vi "sprawdzanie.vi"(5 "String":string, 6 "String 2":string, 7 "String 6":string, 8 "String 3":string, 9 "String 7":string, 10 "String 4":string, 11 "String 8":string, 12 "String 5":string, 13 "String 9":string) -> (18 "X or O":bool, 19 "String 10":string)   [LabVIEW 2023]
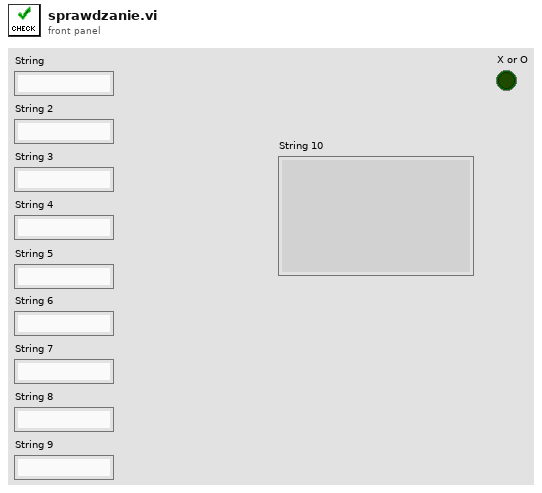
[diagram p1: front panel]
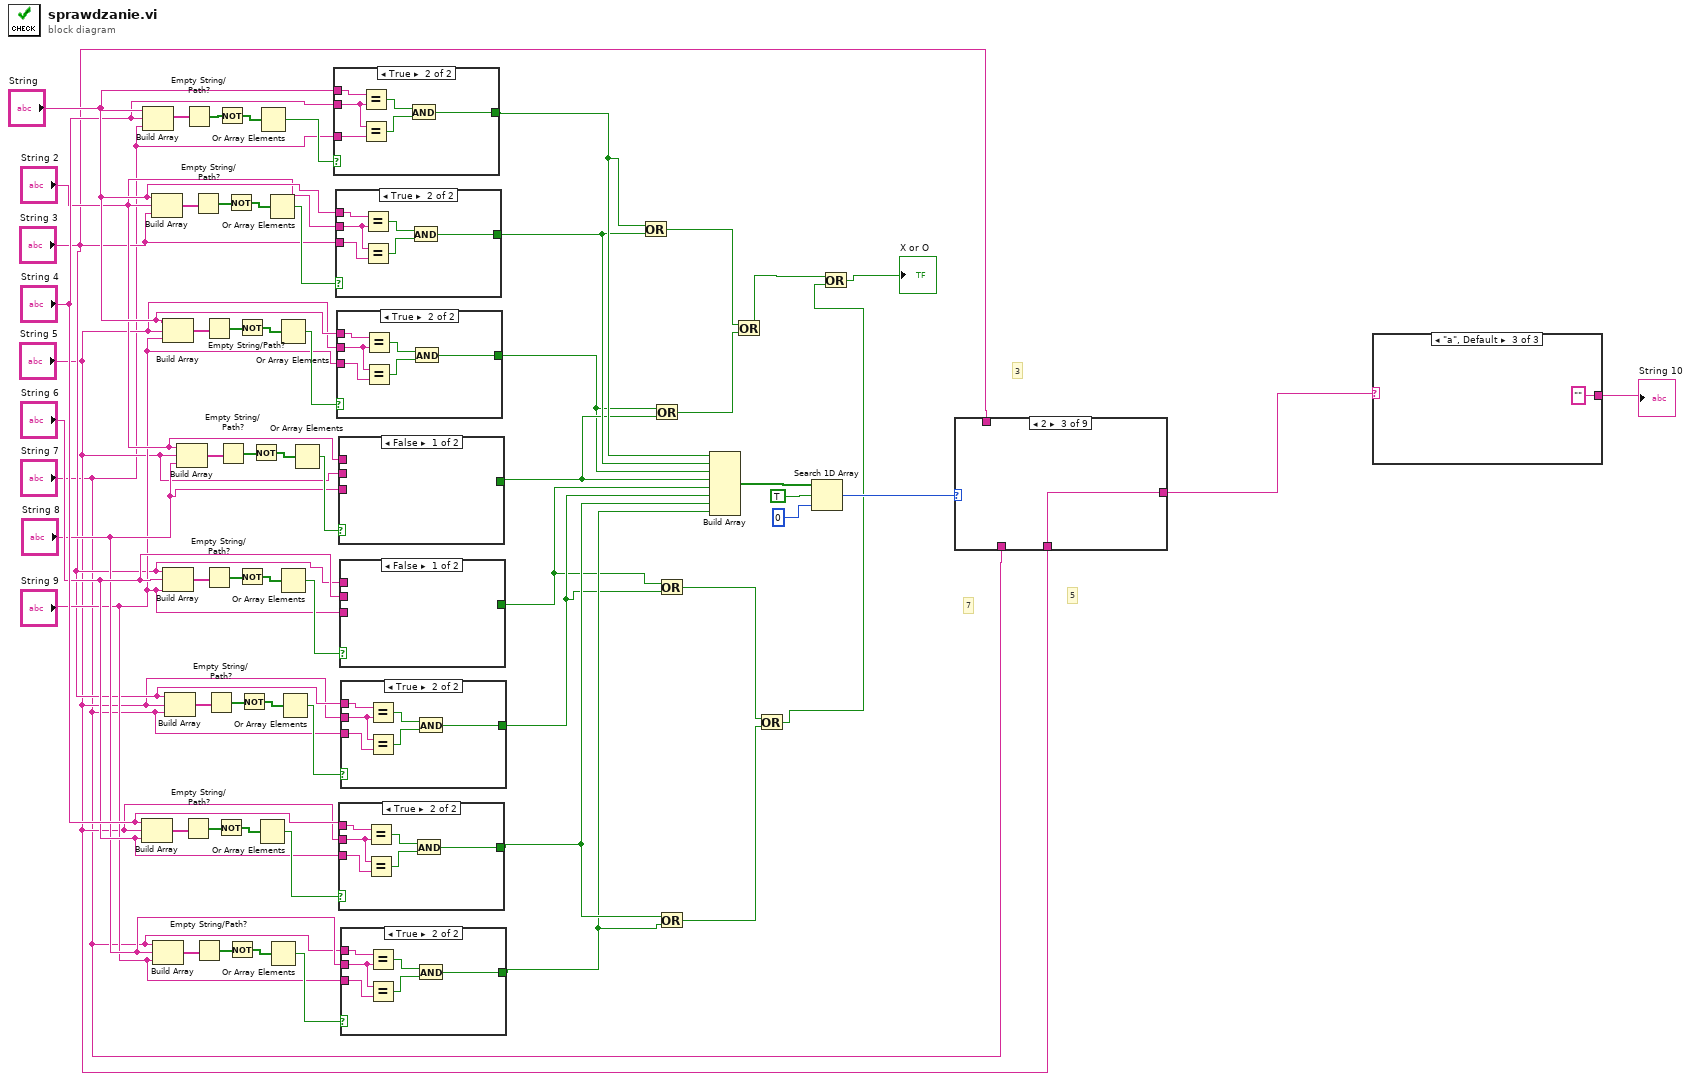
[diagram p0: block diagram]
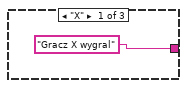
[diagram p2: hidden frame]
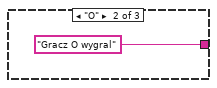
[diagram p3: hidden frame]
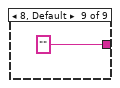
[diagram p11: hidden frame]
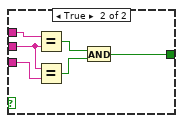
[diagram p15: hidden frame]
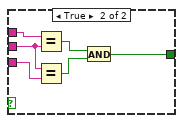
[diagram p16: hidden frame]
diagram:
  # "7"
  # "5"
  # "3"
  n1 = Build Array("String 4", "String 5", "String 6") -> (w36:string[])
  n2 = Build Array("String", "String 4", "String 7") -> (w62:string[])
  n3 = Build Array("String", "String 2", "String 3") -> (w57:string[])
  n4 = Build Array("String 7", "String 8", "String 9") -> (w30:string[])
  n5 = Build Array("String", "String 5", "String 9") -> (w53:string[])
  n6 = Build Array("String 3", "String 6", "String 9") -> (w44:string[])
  n7 = Build Array("String 3", "String 5", "String 7") -> (w40:string[])
  n8 = Build Array("String 2", "String 5", "String 8") -> (w48:string[])
  n9 = Empty String/Path?(string/path=w36) -> (empty?=w35:bool[])
  n10 = Empty String/Path?(string/path=w62) -> (empty?=w61:bool[])
  n11 = Empty String/Path?(string/path=w57) -> (empty?=w56:bool[])
  n12 = Empty String/Path?(string/path=w30) -> (empty?=w29:bool[])
  n13 = Empty String/Path?(string/path=w53) -> (empty?=w54:bool[])
  n14 = Empty String/Path?(string/path=w44) -> (empty?=w43:bool[])
  n15 = Empty String/Path?(string/path=w40) -> (empty?=w39:bool[])
  n16 = Not(x=w35) -> (.not. x?=w37:bool[])
  n17 = Not(x=w61) -> (.not. x?=w59:bool[])
  n18 = Empty String/Path?(string/path=w48) -> (empty?=w47:bool[])
  n19 = Not(x=w56) -> (.not. x?=w58:bool[])
  n20 = Not(x=w29) -> (.not. x?=w31:bool[])
  n21 = Not(x=w54) -> (.not. x?=w52:bool[])
  n22 = Not(x=w43) -> (.not. x?=w45:bool[])
  n23 = Not(x=w39) -> (.not. x?=w41:bool[])
  n24 = Not(x=w47) -> (.not. x?=w49:bool[])
  n25 = Or Array Elements(Boolean array=w37) -> (logical OR=w34:bool)
  n26 = Or Array Elements(Boolean array=w59) -> (logical OR=w60:bool)
  n27 = Or Array Elements(Boolean array=w58) -> (logical OR=w55:bool)
  n28 = Or Array Elements(Boolean array=w31) -> (logical OR=w28:bool)
  n29 = Or Array Elements(Boolean array=w52) -> (logical OR=w51:bool)
  n30 = Or Array Elements(Boolean array=w45) -> (logical OR=w42:bool)
  n31 = Or Array Elements(Boolean array=w41) -> (logical OR=w38:bool)
  n32 = Or Array Elements(Boolean array=w49) -> (logical OR=w46:bool)
  n33 = case shown="True" w60 {
    tunnel: "String" -> [_ w68]
    tunnel: "String 4" -> [_ w66]
    tunnel: "String 7" -> [_ w67]
    tunnel: [_ w63] -> w11
    frame False {
    }
    frame True {
      n34 = Equal?(x=w68, y=w66) -> (x = y?=w65:bool)
      n35 = Equal?(x=w66, y=w67) -> (x = y?=w64:bool)
      n36 = And(x=w65, y=w64) -> (x .and. y?=w63:bool)
    }
  }
  n37 = case shown="True" w55 {
    tunnel: "String" -> [_ w74]
    tunnel: "String 2" -> [_ w72]
    tunnel: "String 3" -> [_ w73]
    tunnel: [_ w69] -> w10
    frame False {
    }
    frame True {
      n38 = Equal?(x=w74, y=w72) -> (x = y?=w71:bool)
      n39 = Equal?(x=w72, y=w73) -> (x = y?=w70:bool)
      n40 = And(x=w71, y=w70) -> (x .and. y?=w69:bool)
    }
  }
  n41 = case shown="True" w51 {
    tunnel: "String" -> [_ w80]
    tunnel: "String 5" -> [_ w78]
    tunnel: "String 9" -> [_ w79]
    tunnel: [_ w75] -> w8
    frame False {
    }
    frame True {
      n42 = Equal?(x=w80, y=w78) -> (x = y?=w77:bool)
      n43 = Equal?(x=w78, y=w79) -> (x = y?=w76:bool)
      n44 = And(x=w77, y=w76) -> (x .and. y?=w75:bool)
    }
  }
  n45 = case shown="False" w46 {
    tunnel: "String 2" -> [_ w86]
    tunnel: "String 5" -> [_ w84]
    tunnel: "String 8" -> [_ w85]
    tunnel: [_ w81] -> w9
    frame False {
    }
    frame True {
      n46 = Equal?(x=w86, y=w84) -> (x = y?=w83:bool)
      n47 = Equal?(x=w84, y=w85) -> (x = y?=w82:bool)
      n48 = And(x=w83, y=w82) -> (x .and. y?=w81:bool)
    }
  }
  n49 = case shown="True" w34 {
    tunnel: "String 4" -> [_ w92]
    tunnel: "String 5" -> [_ w90]
    tunnel: "String 6" -> [_ w91]
    tunnel: [_ w87] -> w17
    frame False {
    }
    frame True {
      n50 = Equal?(x=w92, y=w90) -> (x = y?=w89:bool)
      n51 = Equal?(x=w90, y=w91) -> (x = y?=w88:bool)
      n52 = And(x=w89, y=w88) -> (x .and. y?=w87:bool)
    }
  }
  n53 = case shown="False" w42 {
    tunnel: "String 3" -> [_ w98]
    tunnel: "String 6" -> [_ w96]
    tunnel: "String 9" -> [_ w97]
    tunnel: [_ w93] -> w14
    frame False {
    }
    frame True {
      n54 = Equal?(x=w98, y=w96) -> (x = y?=w95:bool)
      n55 = Equal?(x=w96, y=w97) -> (x = y?=w94:bool)
      n56 = And(x=w95, y=w94) -> (x .and. y?=w93:bool)
    }
  }
  n57 = case shown="True" w38 {
    tunnel: "String 3" -> [_ w104]
    tunnel: "String 5" -> [_ w102]
    tunnel: "String 7" -> [_ w103]
    tunnel: [_ w99] -> w15
    frame False {
    }
    frame True {
      n58 = Equal?(x=w104, y=w102) -> (x = y?=w101:bool)
      n59 = Equal?(x=w102, y=w103) -> (x = y?=w100:bool)
      n60 = And(x=w101, y=w100) -> (x .and. y?=w99:bool)
    }
  }
  n61 = case shown="True" w28 {
    tunnel: "String 7" -> [_ w110]
    tunnel: "String 8" -> [_ w108]
    tunnel: "String 9" -> [_ w109]
    tunnel: [_ w105] -> w16
    frame False {
    }
    frame True {
      n62 = Equal?(x=w110, y=w108) -> (x = y?=w107:bool)
      n63 = Equal?(x=w108, y=w109) -> (x = y?=w106:bool)
      n64 = And(x=w107, y=w106) -> (x .and. y?=w105:bool)
    }
  }
  n65 = Or(x=w11, y=w10) -> (x .or. y?=w7:bool)
  n66 = Or(x=w8, y=w9) -> (x .or. y?=w6:bool)
  n67 = Or(x=w14, y=w15) -> (x .or. y?=w13:bool)
  n68 = Or(x=w17, y=w16) -> (x .or. y?=w12:bool)
  n69 = Build Array(w11, w10, w8, w9, w14, w15, w17, w16) -> (w24:bool[])
  n70 = Or(x=w7, y=w6) -> (x .or. y?=w4:bool)
  n71 = Or(x=w13, y=w12) -> (x .or. y?=w3:bool)
  n72 = Search 1D Array(1D array=w24, element=TRUE, start index (0)=0) -> (index of element=w21:i32)
  n73 = Or(x=w4, y=w3) -> (x .or. y?=→"X or O":bool)
  n74 = case shown="2" w21 {
    tunnel: [w111 w112 w113 w114 w115 w116 w117 w118 "" ("String 10")] -> w2
    tunnel: "String 3" -> [_ w112 _ _ w115 _ _ _ _]
    tunnel: "String 5" -> [_ _ w113 w114 _ w116 w117 _ _]
    tunnel: "String 7" -> [w111 _ _ _ _ _ _ w118 _]
    frame 0 {
    }
    frame 1 {
    }
    frame 2 {
    }
    frame 3 {
    }
    frame 4 {
    }
    frame 5 {
    }
    frame 6 {
    }
    frame 7 {
    }
    frame 8, Default {
    }
  }
  n75 = case shown="\"a\", Default" w2 {
    tunnel: ["Gracz X wygral" ("String 10") "Gracz O wygral" ("String 10") "" ("String 10")] -> w1
    frame "X" {
    }
    frame "O" {
    }
    frame "a", Default {
    }
  }
  "String 10" <- w1
